vi "JSON_TO_Error_description_and_SID.vi"(6 "Sid_present_in_webserver_response":bool, 8 "Error In":errorcluster, 9 "Session id name":string="Sid", 10 "Status code name":string="StatusCode", 11 "JSON String input":string) -> (0 "Error Out":errorcluster, 1 "SID":i32, 2 "status code":i32, 3 "status_selected":string)   [LabVIEW 2017]
doc: "This VI interprets the JSON script and predicts the response from the server\n\nFor ex:\n{\"ErrorCode\":0,\"Sid\":12345}\n\nDisplays:\n0 - \"Success\" All services will respond with this Error Code if there are no errors preventing the web service from being accepted."
panel:
  out "Path of StatusCode ini debug purpose":path
  # "INPUT"
  # "OUTPUT"
  # "ERROR"
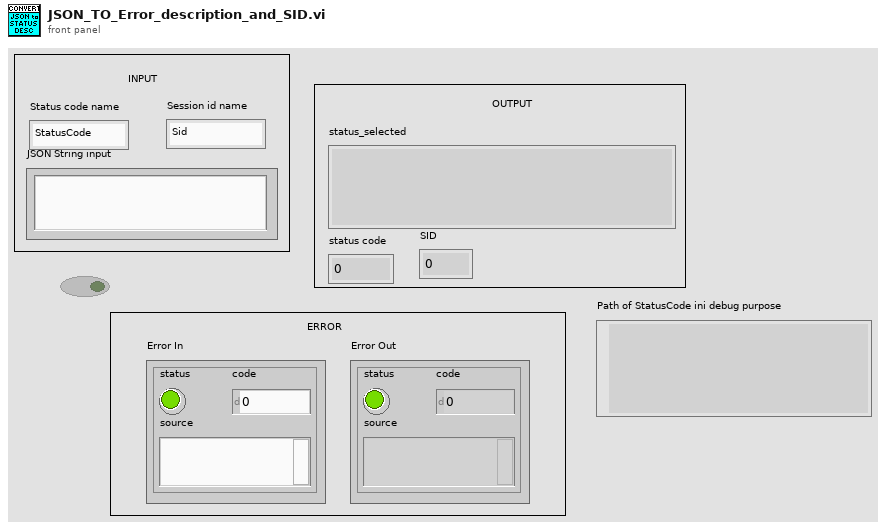
[diagram p1: front panel]
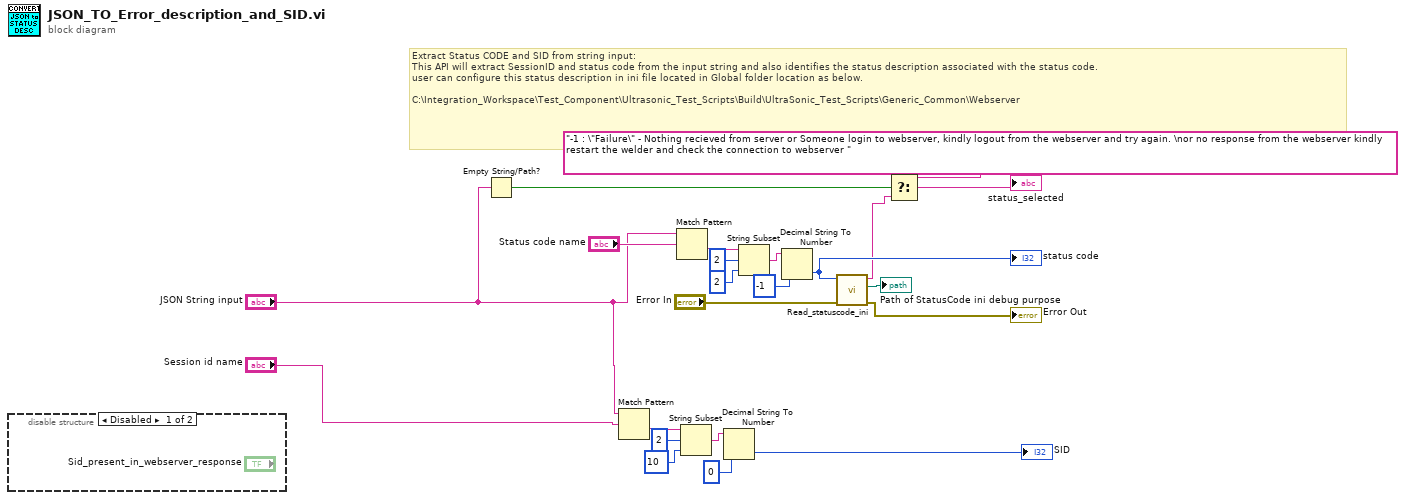
[diagram p0: block diagram]
diagram:
  # "Extract Status CODE and SID from string input:\nThis API will extract SessionID and status code from the input string and also identifies the status description associated with the status code. \nuser can configure this status description in ini file located in Global folder location as below.\n\nC:\\Integration_Workspace\\Test_Component\\Ultrasonic_Test_Scripts\\Build\\UltraSonic_Test_Scripts\\Generic_Common\\Webserver"
  n1 = disable-structure shown="Disabled" {
    frame Disabled {
    }
    frame Enabled {
    }
  }
  n2 = Empty String/Path?(string/path="JSON String input") -> (empty?=w20:bool)
  n3 = Match Pattern(string="JSON String input", regular expression="Session id name") -> (after substring=w10:string)  [unwired: 1 in, 3 out]
  n4 = Match Pattern(string="JSON String input", regular expression="Status code name") -> (after substring=w18:string)  [unwired: 1 in, 3 out]
  n5 = String Subset(string=w10, offset (0)=2, length (rest)=10 ("length (rest)")) -> (substring=w7:string)
  n6 = Decimal String To Number(string=w7, default (0L)=0 ("default (0 I32)")) -> (number=→"SID":i32)  [unwired: 1 in, 1 out]
  n7 = String Subset(string=w18, offset (0)=2, length (rest)=2 ("length (rest)")) -> (substring=w15:string)
  n8 = Decimal String To Number(string=w15, default (0L)=-1 ("default (0 I32)")) -> (number=w12:i32)  [unwired: 1 in, 1 out]
  "status code" <- w12
  n9 = call "Read_statuscode_ini.vi"("Error In"="Error In", "Input status selection"=w12) -> ("Error Out"=→"Error Out":errorcluster, "StatusCode path"=→"Path of StatusCode ini debug purpose":path, "Status_selected"=w11:string)  [unwired: 7 in]
  n10 = Select(t="-1 : \"Failure\" - Nothing recieved from server or Someone login to webserver, kindly logout from the webserver and try again. \nor no response from the webserver kindly restart the welder and check the connection to webserver ", s=w20, f=w11) -> (s? t:f=→"status_selected":string)
